vi "_Remote Set Method Voltages.vi"(6 "use dialog? (F)":bool, 7 "start path":path) -> (0 "error out":errorcluster, 1 "Source/Gas Out":dbl[](array[numeric]), 2 "Voltages":dbl[](array[numeric]))   [LabVIEW 2012]
uses:
  Type/_File Type.ctl
  Type/_RT Active Ch.ctl
  Configuration/_Global Configuration.vi
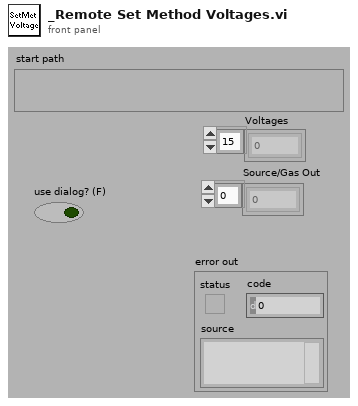
[diagram p1: front panel]
types:
  T1 = typedef "_File Type.ctl" = enum16{"Configuration", "Old Configuration", "Calibration", "Resolution", "Diagnostic Method", "Old Method", "Acq Method", "Samp List"}
  T2 = typedef "_GUI Method.ctl" = cluster{"Lenses":T3[], "Mass Ranges":T4[], "Acquire":bool, "MCA":bool, "Q1DC EN":bool, "Q1 POL":bool, "Q3 POL":bool, "Q1 RF  EN":bool, "Averaging":bool, "Log Scale":bool, "CPS":bool, "Unit":bool, "Data Path":path, "Run Mode":T7, "Fixed Mass (amu)":dbl, "Q3DC EN":bool, "Q3 RF  EN":bool, "Negative":bool}
  T3 = typedef "_Lens Property.ctl" = cluster{"Scan Type":u8, "Scans":i32, "Time 1":dbl, "Time 2":dbl, "Value 1":dbl, "Value 2":dbl, "Step Size":dbl}
  T4 = typedef "_Mass Range Property.ctl" = cluster{"Start":dbl, "Stop":dbl, "Step Size":dbl, "Steps":i32, "Dwell":dbl, "Parameters":T5[], "Res":T6}
  T5 = typedef "_Mass Range Parameters.ctl" = cluster{"Name":string, "Ch#":u8, "StartV":dbl, "StopV":dbl, "StepV":dbl, "Index":u8}
  T6 = typedef "_RT Res Type.ctl" = u16
  T7 = typedef "_Run Mode.ctl" = enum16{"MRM (Q1/Q2)", "Q1 Scan", "Q1 SRM", "Q2 Scan", "Q2 SRM", "Product Scan", "Precursor Scan", "Neutral Loss", "Neutral Gain"}
  T8 = typedef "_RT Instrument 2.ctl" = cluster{"Table":T9[], "Instrument":string[]}
  T9 = typedef "_RT Configuration 2.ctl" = cluster{"Name":string, "Ch#":u8, "Min":dbl, "Max":dbl, "Def+":dbl, "Def-":dbl, "Offset":dbl, "Slope":dbl, "Type":u8, "Description":string, "SettleT":dbl}
  T10 = typedef "_RT Active Ch.ctl" = cluster{"Start":i32, "Step":i32, "ChID":i32}
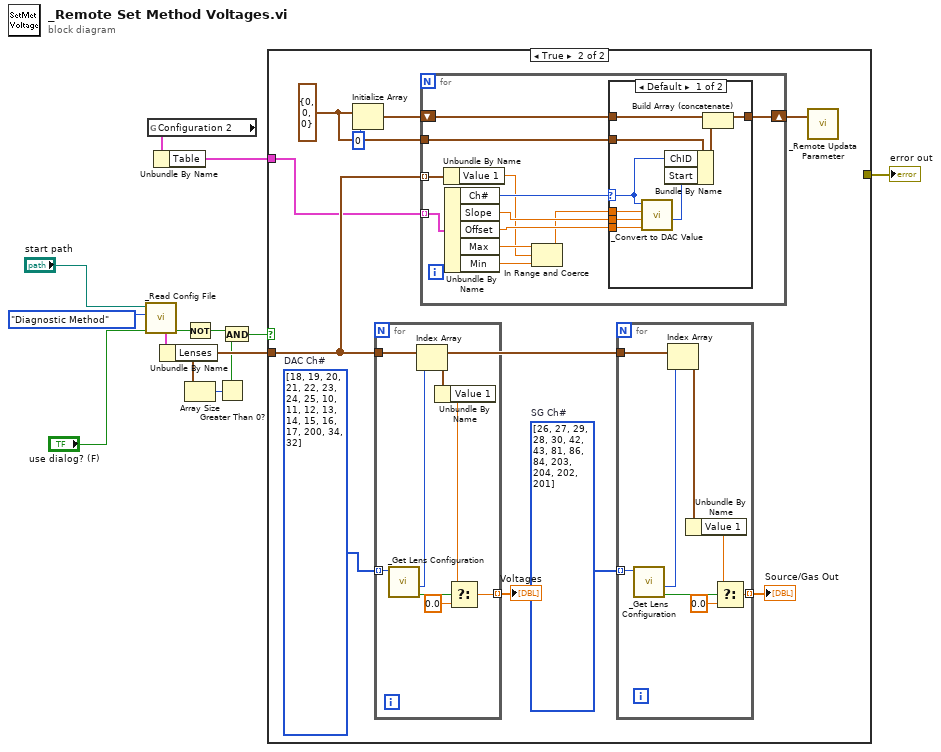
[diagram p0: block diagram]
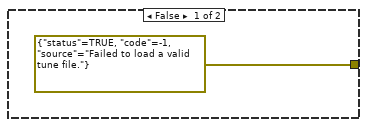
[diagram p2: hidden frame]
diagram:
  n1 = call "_Read Config File.vi"("advisory dialog? (display:T)"="use dialog? (F)", "File Type (config)"=_File_Type."Diagnostic Method", "start path  (Not A Path)"="start path") -> ("error"=w6:bool, "GUI Method"=w12:T2)  [unwired: 7 out]
  n2 = global read "_Global Configuration.vi" "Configuration 2"() -> (w9:T8)
  n3 = Unbundle By Name(w9) -> ("Table"=w8:T9[])
  n4 = Unbundle By Name(w12) -> ("Lenses"=w11:T3[])
  n5 = Not(x=w6) -> (.not. x?=w5:bool)
  n6 = Array Size(array=w11) -> (size(s)=w10:i32)
  n7 = Greater Than 0?(x=w10) -> (x > 0?=w4:bool)
  n8 = And(x=w5, y=w4) -> (x .and. y?=w3:bool)
  n9 = case shown="True" w3 {
    tunnel: w11 -> [_ w20]
    tunnel: w8 -> [_ w19]
    tunnel: [errorcluster {"status"=TRUE, "code"=-1, "source"="Failed to load a valid tune file."} ("error out") _] -> w7
    frame False {
    }
    frame True {
      w16 = T10 {"Start"=0, "Step"=0, "ChID"=0} ("Active Channel")
      w22 = u8[] [26, 27, 29, 28, 30, 42, 43, 81, 86, 84, 203, 204, 202, 201]  # SG Ch#
      w24 = u8[] [18, 19, 20, 21, 22, 23, 24, 25, 10, 11, 12, 13, 14, 15, 16, 17, 200, 34, 32]  # DAC Ch#
      n10 = Initialize Array(w16, 0 ("dimension size")) -> (w17:T10[])
      n11 = for {
        tunnel: w24 -> [w62] mode=indexing
        tunnel: [w55] -> w23 mode=indexing
        tunnel: w20 -> [w61]
        n12 = call "_Get Lens Configuration.vi"("Channel #"=w62) -> ("Found"=w58:bool, "Config Row#"=w60:i32)  [unwired: 1 in, 4 out]
        n13 = Index Array(array=w61, index=w60) -> (element=w59:T3)
        n14 = Unbundle By Name(w59) -> ("Value 1"=w57:dbl)
        n15 = Select(t=w57, s=w58, f=0.0) -> (s? t:f=w55:dbl)
      }
      "Voltages" <- w23
      n16 = for {
        tunnel: w19 -> [w33] mode=indexing
        tunnel: w20 -> [w32] mode=indexing
        shift-right: [w30] -> w15
        shift-left: w17 -> [w31]
        tunnel: w16 -> [w29]
        n17 = Unbundle By Name(w32) -> ("Value 1"=w26:dbl)
        n18 = Unbundle By Name(w33) -> ("Ch#"=w34:u8, "Slope"=w36:dbl, "Offset"=w35:dbl, "Max"=w28:dbl, "Min"=w27:dbl)
        n19 = In Range and Coerce(upper limit=w28, x=w26, lower limit=w27) -> (coerced(x)=w25:dbl)  [unwired: 1 out]
        n20 = case shown="Default" w34 {
          selector: w34 -> [w41 _]
          tunnel: w25 -> [w45 _]
          tunnel: w36 -> [w44 _]
          tunnel: w35 -> [w43 _]
          tunnel: w31 -> [w42 w46]
          tunnel: [w37 w46] -> w30
          tunnel: w29 -> [w39 _]
          frame Default {
            n21 = call "_Convert to DAC Value.vi"("Offset"=w43, "Slop"=w44, "Number"=w45, "Channel"=w41) -> ("DAC Value"=w40:i32)  [unwired: 2 in, 5 out]
            n22 = Bundle By Name(cluster=w39, "ChID"=w41, "Start"=w40) -> (w38:T10)
            n23 = Build Array (concatenate)(w42, w38) -> (w37:T10[])
          }
          frame 0..2, 4, 5, 7, 9 {
            # "skip mass & PW\nchannels"
          }
        }
      }
      n24 = for {
        tunnel: w22 -> [w54] mode=indexing
        tunnel: [w47] -> w21 mode=indexing
        tunnel: w20 -> [w52]
        n25 = call "_Get Lens Configuration.vi"("Channel #"=w54) -> ("Found"=w49:bool, "Config Row#"=w51:i32)  [unwired: 1 in, 4 out]
        n26 = Index Array(array=w52, index=w51) -> (element=w53:T3)
        n27 = Unbundle By Name(w53) -> ("Value 1"=w48:dbl)
        n28 = Select(t=w48, s=w49, f=0.0) -> (s? t:f=w47:dbl)
      }
      "Source/Gas Out" <- w21
      n29 = call "_Remote Updata Parameter.vi"("Parameters"=w15) -> ()  [unwired: 1 in, 1 out]
    }
  }
  "error out" <- w7
